vi "Player Info.vi"(11 "Class":refnum<class "Pinwheel.lvclass">) -> (0 "Defeat Speech":string, 1 "Victory Speech":string, 2 "Name":string, 3 "Class":refnum<class "Pinwheel.lvclass">)   [LabVIEW 2015, in "Pinwheel.lvclass"]
uses:
  Pinwheel.lvclass
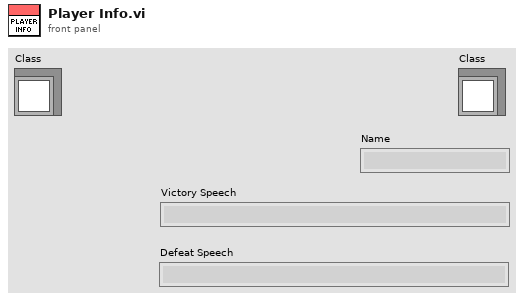
[diagram p1: front panel]
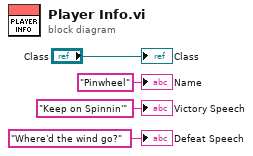
[diagram p0: block diagram]
diagram:
  "Class" <- "Class"
  "Name" <- "Pinwheel" ("Name")
  "Victory Speech" <- "Keep on Spinnin'" ("Victory Speech")
  "Defeat Speech" <- "Where'd the wind go?" ("Defeat Speech")
